vi "SecondaryRobotFunctions.vi"(6 "Robot State":T1, 7 "Automatic State Control Mode (F)":bool, 8 "Secondary Joystick Values":dbl[](array[numeric]), 9 "ADIS Gyro Values":T12 {"IMU Data Out"."X Accel (g)" format="%#_3g"; "IMU Data Out"."Y Accel (g)" format="%#_3g"; "IMU Data Out"."Z Accel (g)" format="%#_3g"}, 10 "Drive Joystick Buttons":bool[](array[boolean]), 11 "Secondary Joystick Buttons":bool[](array[boolean])) -> ()   [LabVIEW 2018]
uses:
  Controls/ADIS Gyro Values.ctl
  Controls/Robot State.ctl
  Controls/Robot Pivot Motion Commands.ctl
  Controls/Pivot Motor Commands.ctl
  Controls/Robot Drive Mode.ctl
  Controls/Climb Motor Commands.ctl
  Controls/Arm Motor Commands.ctl
  Controls/Ball Motor Commands.ctl
  Controls/Dics Eject Command.ctl
  Controls/Lift Motor Commands.ctl
  Controls/Grip Motor Commands.ctl
  Controls/Enable Actions.ctl
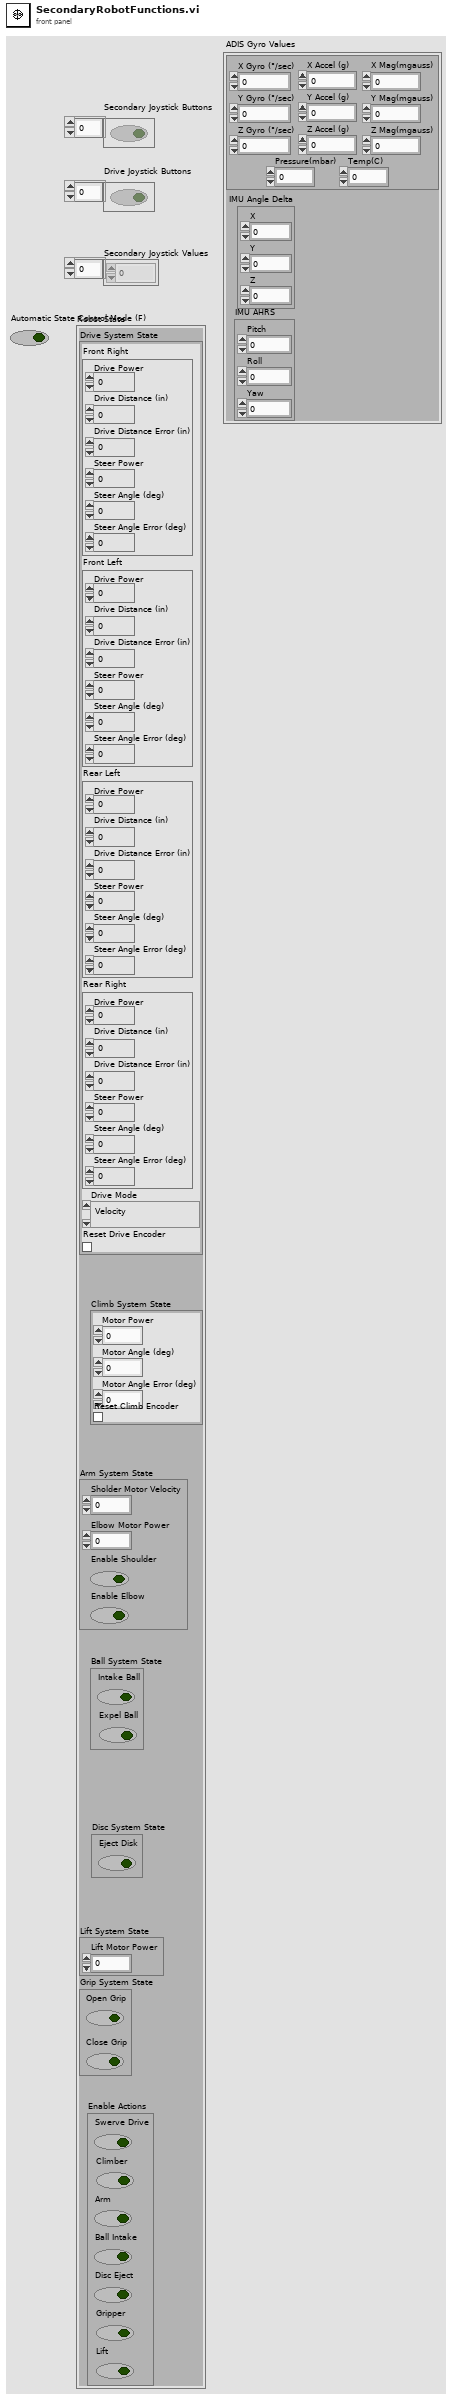
[diagram p1: front panel]
types:
  T1 = typedef "Robot State.ctl" = cluster{"Drive System State":T2, "Climb System State":T5, "Arm System State":T6, "Ball System State":T7, "Disc System State":T8, "Lift System State":T9, "Grip System State":T10, "Enable Actions":T11}
  T2 = typedef "Robot Pivot Motion Commands.ctl" = cluster{"Front Right":T3, "Front Left":T3, "Rear Left":T3, "Rear Right":T3, "Drive Mode":T4, "Reset Drive Encoder":bool}
  T3 = typedef "Pivot Motor Commands.ctl" = cluster{"Drive Power":dbl, "Drive Distance (in)":dbl, "Drive Distance Error (in)":dbl, "Steer Power":dbl, "Steer Angle (deg)":dbl, "Steer Angle Error (deg)":dbl}
  T4 = typedef "Robot Drive Mode.ctl" = enum16{"Velocity", "Distance"}
  T5 = typedef "Climb Motor Commands.ctl" = cluster{"Motor Power":dbl, "Motor Angle (deg)":dbl, "Motor Angle Error (deg)":dbl, "Reset Climb Encoder":bool}
  T6 = typedef "Arm Motor Commands.ctl" = cluster{"Enable Shoulder":bool, "Enable Elbow":bool, "Elbow Motor Power":dbl, "Sholder Motor Velocity":dbl}
  T7 = typedef "Ball Motor Commands.ctl" = cluster{"Intake Ball":bool, "Expel Ball":bool}
  T8 = typedef "Dics Eject Command.ctl" = cluster{"Eject Disk":bool}
  T9 = typedef "Lift Motor Commands.ctl" = cluster{"Lift Motor Power":dbl}
  T10 = typedef "Grip Motor Commands.ctl" = cluster{"Open Grip":bool, "Close Grip":bool}
  T11 = typedef "Enable Actions.ctl" = cluster{"Swerve Drive":bool, "Climber":bool, "Arm":bool, "Ball Intake":bool, "Disc Eject":bool, "Gripper":bool, "Lift":bool}
  T12 = typedef "ADIS Gyro Values.ctl" = cluster{"IMU Data Out":cluster{"X Gyro (°/sec)":dbl, "Y Gyro (°/sec)":dbl, "Z Gyro (°/sec)":dbl, "X Accel (g)":dbl, "Y Accel (g)":dbl, "Z Accel (g)":dbl, "X Mag(mgauss)":dbl, "Y Mag(mgauss)":dbl, "Z Mag(mgauss)":dbl, "Pressure(mbar)":dbl, "Temp(C)":dbl}, "IMU Angle Delta":cluster{"X":dbl, "Y":dbl, "Z":dbl}, "IMU AHRS":cluster{"Pitch":dbl, "Roll":dbl, "Yaw":dbl}}
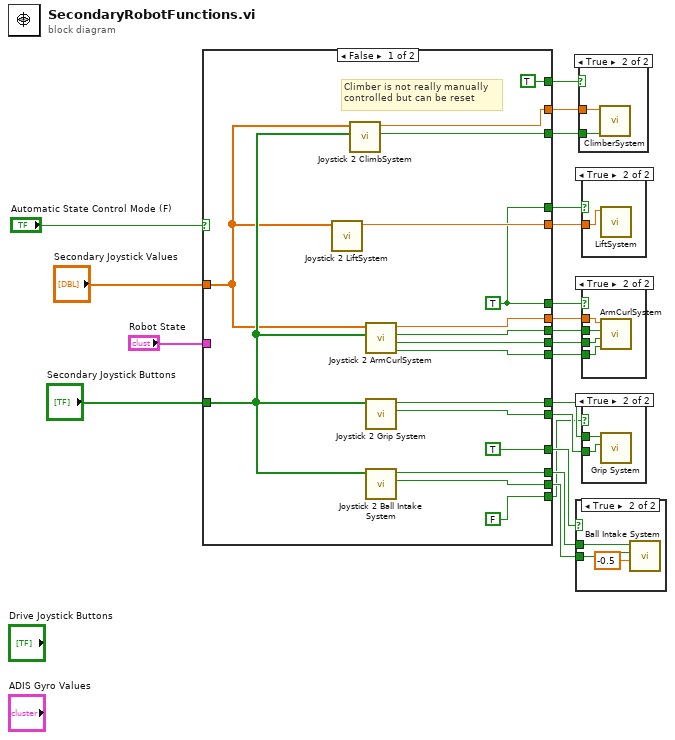
[diagram p0: block diagram]
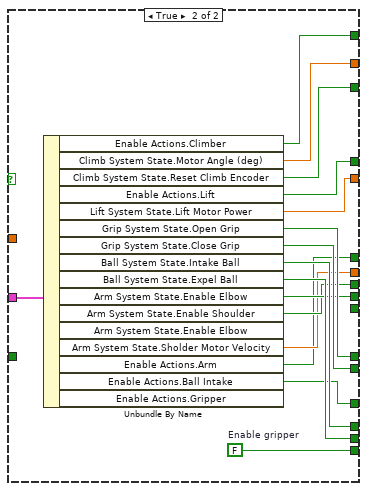
[diagram p6: hidden frame]
diagram:
  n1 = case shown="False" "Automatic State Control Mode (F)" {
    tunnel: "Secondary Joystick Buttons" -> [w24 _]
    tunnel: [w37 w46] -> w19
    tunnel: [w36 w47] -> w18
    tunnel: [w35 w48] -> w17
    tunnel: [w34 _] -> w16
    tunnel: "Secondary Joystick Values" -> [w23 _]
    tunnel: [w33 w50] -> w14
    tunnel: [w32 w49] -> w13
    tunnel: [w31 w42] -> w12
    tunnel: [w30 w53] -> w7
    tunnel: [w29 w51] -> w11
    tunnel: "Robot State" -> [_ w52]
    tunnel: [w28 w41] -> w8
    tunnel: [w28 w45] -> w6
    tunnel: [TRUE ("Ball Intake") w44] -> w5
    tunnel: [FALSE w43] -> w4
    tunnel: [w21 w40] -> w3
    tunnel: [w22 w39] -> w2
    tunnel: [TRUE ("Climber") w38] -> w1
    frame False {
      w28 = TRUE ("Lift")
      # "Climber is not really manually\ncontrolled but can be reset"
      n2 = call "Joystick 2 LiftSystem.vi"("JoystickAxes"=w23) -> ("Lift Speed"=w31:dbl)  [unwired: 10 in]
      n3 = call "Joystick 2 ClimbSystem.vi"("Secondary Joystick Buttons"=w24, "Secondary Joystick Values"=w23) -> ("Reset Climber Encoder"=w22:bool, "Desired Climber Angle"=w21:dbl)  [unwired: 8 in]
      n4 = call "Joystick 2 ArmCurlSystem.vi"("Secondary Joystick Buttons"=w24, "Secondary Joystick Values"=w23) -> ("Reset Arm Encoders"=w34:bool, "ElbowMotor"=w35:bool, "ShoulderMotor"=w36:bool, "Curl Speed"=w37:dbl)  [unwired: 6 in]
      n5 = call "Joystick 2 Grip System.vi"("Secondary joystick buttons"=w24) -> ("Close Grip"=w29:bool, "Open Grip"=w30:bool)  [unwired: 9 in]
      n6 = call "Joystick 2 Ball Intake System.vi"("Secondary Joystick Buttons"=w24) -> ("Outtake"=w32:bool, "Intake"=w33:bool)  [unwired: 9 in]
    }
    frame True {
      w43 = FALSE  # Enable gripper
      n7 = Unbundle By Name(w52) -> ("Enable Actions.Climber"=w38:bool, "Climb System State.Motor Angle (deg)"=w40:dbl, "Climb System State.Reset Climb Encoder"=w39:bool, "Enable Actions.Lift"=w41:bool, "Lift System State.Lift Motor Power"=w42:dbl, "Grip System State.Open Grip"=w53:bool, "Grip System State.Close Grip"=w51:bool, "Ball System State.Intake Ball"=w50:bool, "Ball System State.Expel Ball"=w49:bool, "Arm System State.Enable Elbow"=w48:bool, "Arm System State.Enable Shoulder"=w47:bool, "Arm System State.Sholder Motor Velocity"=w46:dbl, "Enable Actions.Arm"=w45:bool, "Enable Actions.Ball Intake"=w44:bool)  [unwired: 2 out]
    }
  }
  n8 = case shown="True" w5 {
    tunnel: w14 -> [_ w56]
    tunnel: w13 -> [_ w55]
    frame False {
    }
    frame True {
      n9 = call "Ball Intake System.vi"("Scaling factor"=-0.5, "Outtake"=w55, "Intake"=w56) -> ()  [unwired: 9 in]
    }
  }
  n10 = case shown="True" w1 {
    tunnel: w3 -> [_ w58]
    tunnel: w2 -> [_ w57]
    frame False {
    }
    frame True {
      n11 = call "ClimberSystem.vi"("Reset Climb Encoder"=w57, "Desired Angle (deg)"=w58) -> ()  [unwired: 10 in]
    }
  }
  n12 = case shown="True" w8 {
    tunnel: w12 -> [_ w59]
    frame False {
    }
    frame True {
      n13 = call "LiftSystem.vi"("Lift Speed"=w59) -> ()  [unwired: 11 in]
    }
  }
  n14 = case shown="True" w6 {
    tunnel: w19 -> [_ w63]
    tunnel: w18 -> [_ w62]
    tunnel: w17 -> [_ w61]
    tunnel: w16 -> [_ w60]
    frame False {
    }
    frame True {
      n15 = call "ArmCurlSystem.vi"("Reset Encoder"=w60, "Elbow Motor"=w61, "Shoulder Motor"=w62, "Curl Speed"=w63) -> ()  [unwired: 8 in]
    }
  }
  n16 = case shown="True" w4 {
    tunnel: w7 -> [_ w65]
    tunnel: w11 -> [_ w64]
    frame False {
    }
    frame True {
      n17 = call "Grip System.vi"("Close Grip"=w64, "Open Grip"=w65) -> ()  [unwired: 10 in]
    }
  }
